vi "ma_catch.vi"(8 "Error":errorcluster, 11 "KNR in":T2) -> (0 "error out 4":errorcluster caption="error out", 1 "Number of Matches (Shape Detection 1)":i32, 2 "Circles (Shape Detection 1)":T1(array[cluster]) {"Position"."Y" format="%.2f"; "Position"."X" format="%.2f"}, 3 "KNR out":T2, 5 "配對積木":bool[][](array[boolean]), 7 "配對數":i32)   [LabVIEW 2013]
uses:
  <userlib>/KNR OS 3.0 LabVIEW Toolkit/Type Definition/KNR3 Reference.ctl
  <userlib>/_FPGA Interface Advanced Tools/FPGA Interface Base/FPGA Interface Base.lvclass
  <userlib>/KNR OS 3.0 LabVIEW Toolkit/Type Definition/Resource.ctl
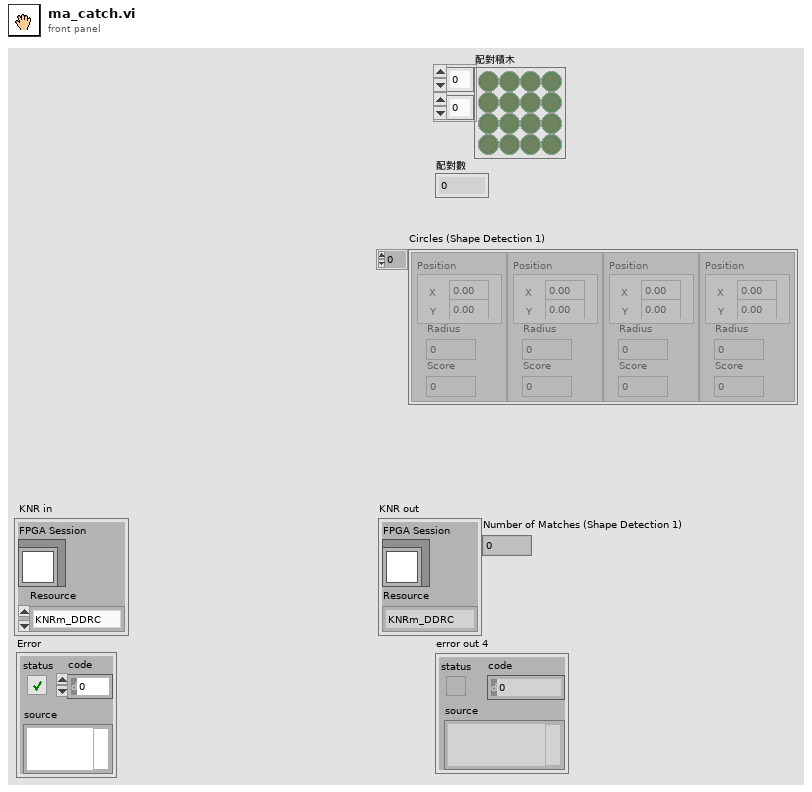
[diagram p1: front panel]
types:
  T1 = cluster{"Position":cluster{"X":sgl, "Y":sgl}, "Radius":dbl, "Score":dbl}[]
  T2 = typedef "KNR3 Reference.ctl" = cluster{"FPGA Session":refnum<class "FPGA Interface Base.lvclass">, "Resource":T3}
  T3 = typedef "Resource.ctl" = enum16{"KNRm_DDRC", "KNRm_DDDD", "KNRm_DDDR", "KNRm_DDDC", "KNR"}
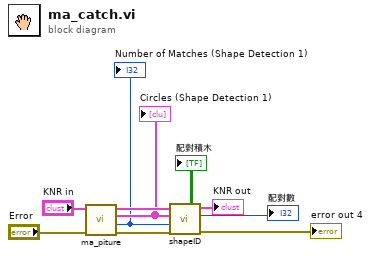
[diagram p0: block diagram]
diagram:
  n1 = call "ma_piture.vi"("Error"="Error", "KNR in"="KNR in") -> ("error out"=w7:errorcluster, "Number of Matches (Shape Detection 1)"=w8:i32, "Circles (Shape Detection 1)"=w9:T1, "KNR out"=w10:T2)  [unwired: 5 in, 1 out]
  "Circles (Shape Detection 1)" <- w9
  "Number of Matches (Shape Detection 1)" <- w8
  n2 = call "shapeID.vi"("Error"=w7, "Nb Circles (Circle Detection 1)"=w8, "Circles (Shape Detection 1)"=w9, "KNR in"=w10) -> ("error out 4"=→"error out 4":errorcluster, "配對數"=→"配對數":i32, "KNR out"=→"KNR out":T2, "配對積木"=→"配對積木":bool[][])  [unwired: 4 in]
